vi "Fill Tank C.vi"() -> ()   [LabVIEW 2018]
panel:
  in  "fill tank C -\nvalve 12 open":bool[](array[boolean])=[TRUE, TRUE, FALSE, FALSE, TRUE, TRUE, FALSE, FALSE, TRUE, FALSE, FALSE, FALSE]
  out "error out":errorcluster
  in  "error in (no error)":errorcluster
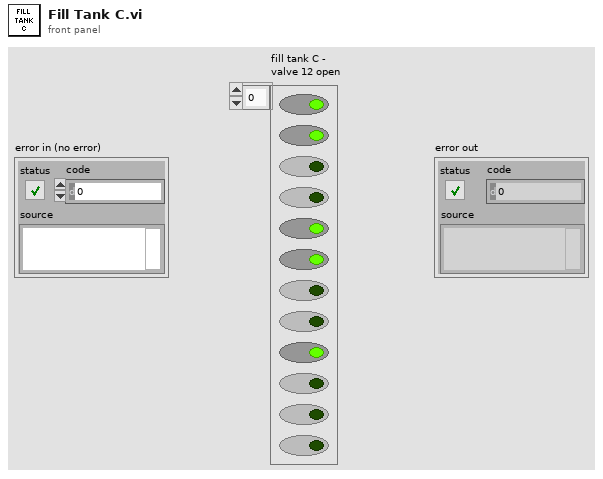
[diagram p1: front panel]
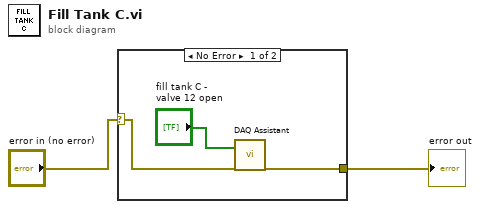
[diagram p0: block diagram]
diagram:
  n1 = case shown="No Error" "error in (no error)" {
    selector: "error in (no error)" -> [w3 w6]
    tunnel: [w4 w6] -> w2
    frame No Error {
      n2 = call "DAQ Assistant"("data"="fill tank C -\nvalve 12 open", "error in"=w3) -> ("error out"=w4:errorcluster)  [unwired: 16 in, 1 out]
    }
    frame Error {
    }
  }
  "error out" <- w2
